vi "ge_CnvrtString2Enum.vi"(8 "error in (no error)":errorcluster, 11 "Enum String":string) -> (0 "error out":errorcluster, 3 "Hdr Name":T1)   [LabVIEW 2012]
uses:
  Common/Controls/HeaderNames.ctl
  <vilib>/Utility/VariantDataType/VariantType.lvlib
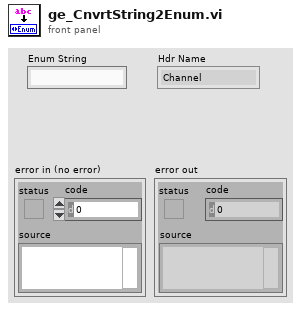
[diagram p1: front panel]
types:
  T1 = typedef "HeaderNames.ctl" = enum16{"Channel", "Device", "Spacer", "Description", "MB", "Range", "Terminal", "Coupling", "Thresh (V)", "Pulse/Rev", "Slope", "Min EU", "Min RPM", "mV/EU", "Iex", "Temp Units", "Type", "CJC Src", "CJC Val", "Ro", "Wire Cfg", "Strain Mode", "Vex", "Bridge Type", "GF", "Gauge Res", "Poisson", "Lead Res", "Init Strain", "GAF", "Scale", "Offset", "Unit (EU)", "dB?", "dB Ref", "Cal Mag", "Cal Units", "Max Temp", "Min Temp", "Max Strain", "Min Strain"}
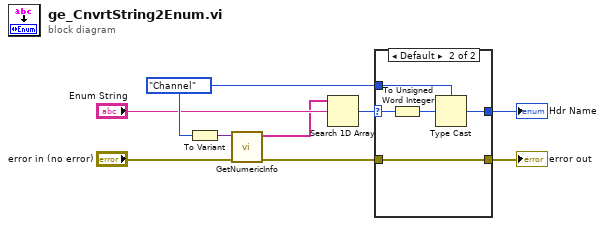
[diagram p0: block diagram]
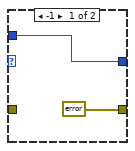
[diagram p2: hidden frame]
diagram:
  w8 = HeaderNames."Channel" ("Hdr Name")
  n1 = To Variant(anything=w8) -> (Variant=w5:variant)
  n2 = call <vilib>:"GetNumericInfo.vi"("error in (no error)"="error in (no error)", "Variant"=w5) -> ("error out"=w2:errorcluster, "EnumNames"=w6:string[])  [unwired: 6 in, 2 out]
  n3 = Search 1D Array(1D array=w6, element="Enum String") -> (index of element=w3:i32)  [unwired: 1 in]
  n4 = case shown="Default" w3 {
    selector: w3 -> [_ w13]
    tunnel: [w11 w16] -> w9
    tunnel: w8 -> [w11 w15]
    tunnel: w2 -> [_ w12]
    tunnel: [errorcluster {"status"=TRUE, "code"=5000, "source"="ge_CnvrtString2Enum.vi<ERR>String value is not defined by the enum type def."} ("error out") w12] -> w1
    frame -1 {
    }
    frame Default {
      n5 = To Unsigned Word Integer(number=w13) -> (unsigned 16bit integer=w14:u16)
      n6 = Type Cast(type=w15, x=w14) -> (*(type *) &x=w16:T1)
    }
  }
  "Hdr Name" <- w9
  "error out" <- w1
